vi "Save Class Library.vi"(8 "Error In":errorcluster, 11 "Library Ref in":refnum<vi>) -> (0 "Error Out":errorcluster)   [LabVIEW 2013, in "Scripter.lvlib"]
uses:
  Scripter.lvlib
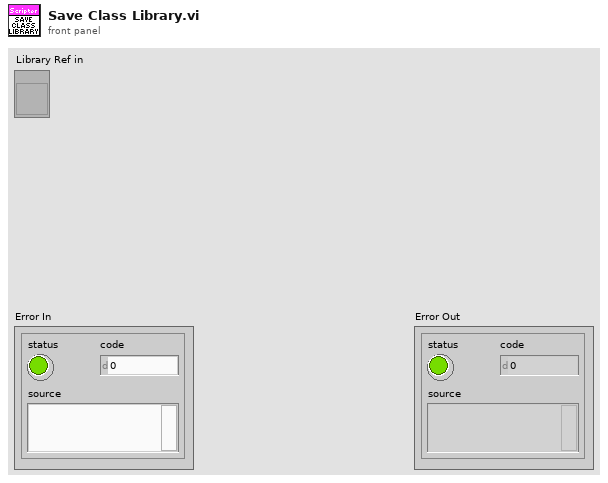
[diagram p1: front panel]
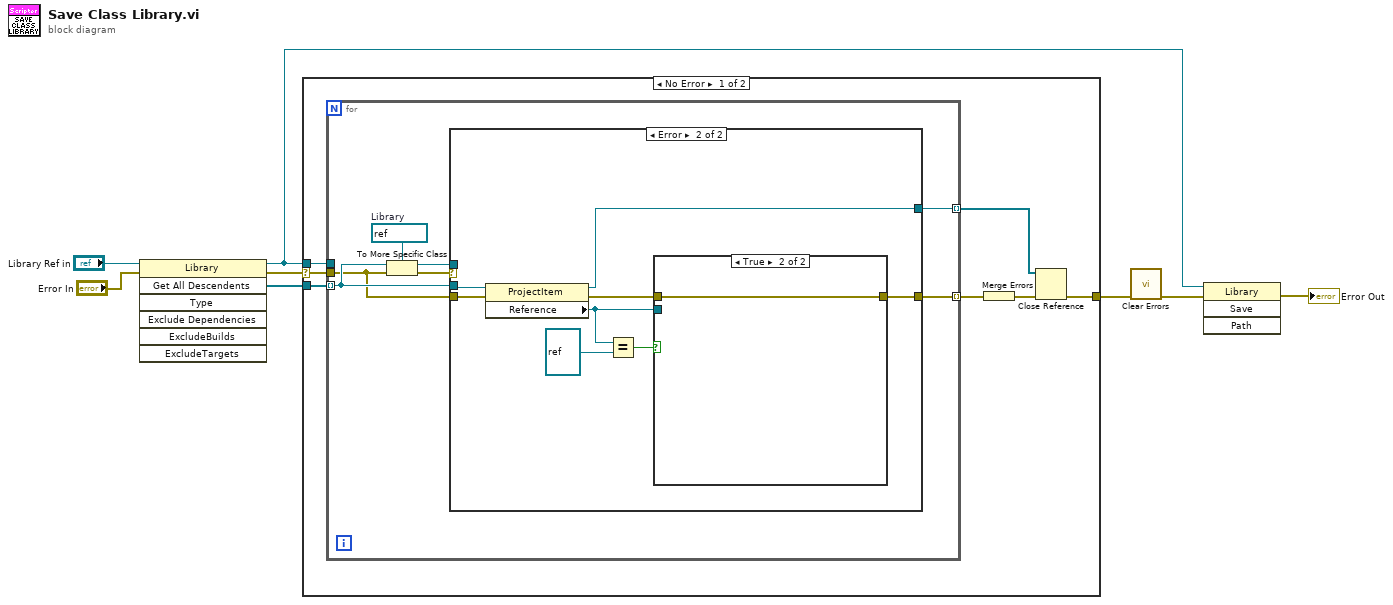
[diagram p0: block diagram]
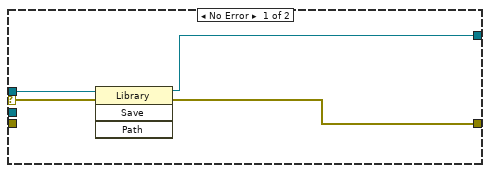
[diagram p2: hidden frame]
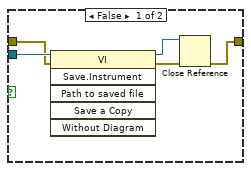
[diagram p3: hidden frame]
diagram:
  n1 = invoke class="Library" method="Get All Descendents"(reference="Library Ref in", error in="Error In") -> (reference out=w2:refnum<vi>, error out=w5:errorcluster, "All Descendents"=w7:refnum<vi>[])  [unwired: 5 in, 4 out]
  n2 = case shown="No Error" w5 {
    selector: w5 -> [w14 w41]
    tunnel: w7 -> [w15 _]
    tunnel: w2 -> [w13 _]
    tunnel: [w9 w41] -> w4
    frame No Error {
      n3 = for {
        tunnel: w15 -> [w19] mode=indexing
        tunnel: w14 -> [w18]
        tunnel: w13 -> [_]
        tunnel: [w17] -> w12 mode=indexing
        tunnel: [w16] -> w10 mode=indexing
        w22 = refnum<vi> refnum  # Library
        n4 = To More Specific Class(target class=w22, reference=w19, error in=w18) -> (specific class reference=w20:refnum<vi>, error out=w21:errorcluster)
        n5 = case shown="Error" w21 {
          selector: w21 -> [w24 _]
          tunnel: w20 -> [w26 _]
          tunnel: w19 -> [_ w34]
          tunnel: w18 -> [_ w30]
          tunnel: [w25 w28] -> w16
          tunnel: [w23 w27] -> w17
          frame No Error {
            n6 = invoke class="Library" method="Save"(reference=w26, error in=w24) -> (reference out=w25:refnum<vi>, error out=w23:errorcluster)  [unwired: 2 in, 2 out]
          }
          frame Error {
            n7 = property class="ProjectItem"(reference=w34, error in=w30) -> (reference out=w28:refnum<vi>, error out=w29:errorcluster, "Reference"=w31:refnum<vi>)
            n8 = Equal?(x=w31, y=refnum<vi> refnum) -> (x = y?=w32:bool)
            n9 = case shown="True" w32 {
              tunnel: w31 -> [w39 _]
              tunnel: w29 -> [w36 w40]
              tunnel: [w35 w40] -> w27
              frame False {
                n10 = invoke class="VI" method="Save.Instrument"(reference=w39, error in=w36) -> (reference out=w37:refnum<vi>, error out=w38:errorcluster)  [unwired: 4 in, 4 out]
                n11 = Close Reference(reference=w37, error in (no error)=w38) -> (error out=w35:errorcluster)
              }
              frame True {
              }
            }
          }
        }
      }
      n12 = Merge Errors(w12) -> (w11:errorcluster)
      n13 = Close Reference(reference=w10, error in (no error)=w11) -> (error out=w9:errorcluster)
    }
    frame Error {
    }
  }
  n14 = call <vilib>:"Clear Errors.vi"("error in (no error)"=w4) -> ("error out"=w3:errorcluster)  [unwired: 6 in]
  n15 = invoke class="Library" method="Save"(reference=w2, error in=w3) -> (error out=→"Error Out":errorcluster)  [unwired: 2 in, 3 out]
